vi "BIN_PAQ_UpdateIndexFile.vi"(8 "error in (no error)":errorcluster, 10 "path":path, 11 "TimeRange":T1) -> (0 "error out":errorcluster)   [LabVIEW 2020, in "Sgraph_lib_V1.lvlib" / "DBAL-BIN.lvclass"]
doc: "This method performs a 'read-modify-write' action on the index file that belongs to this table type.\nOnly the line is updated that belongs to the sequence number of this PAQ file.\n\nThe index file enables fast readback for finding the correct file sequence number."
uses:
  DBAL-BIN.lvclass
  controls/DBAL_PAQ_TimeRange.ctl
  DBAL.lvclass
panel:
  out "FileName":string
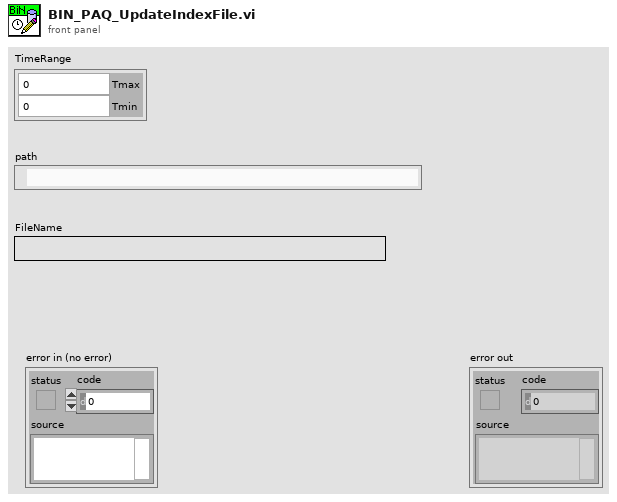
[diagram p1: front panel]
types:
  T1 = typedef "Sgraph_lib_V1.lvlib/DBAL.lvclass/DBAL_PAQ_TimeRange.ctl" = cluster{"Tmax":dbl, "Tmin":dbl}
  T2 = enum16{"open", "replace", "create", "open or create", "replace or create", "replace or create with confirmation"}
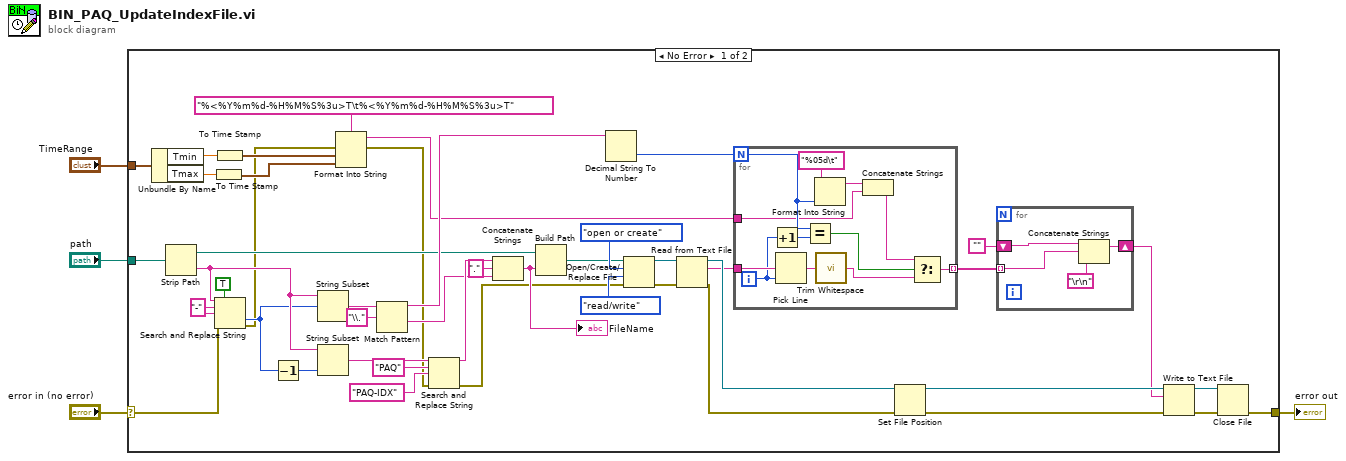
[diagram p0: block diagram]
diagram:
  n1 = case shown="No Error" "error in (no error)" {
    selector: "error in (no error)" -> [w47 w66]
    tunnel: [w19 w66] -> w3
    tunnel: "TimeRange" -> [w15 _]
    tunnel: "path" -> [w49 _]
    frame No Error {
      w48 = "-" ("search string")
      n2 = Unbundle By Name(w15) -> ("Tmin"=w13:dbl, "Tmax"=w14:dbl)
      n3 = Strip Path(path=w49) -> (stripped path=w33:path, name=w45:string)
      n4 = To Time Stamp(1:w14) -> (0:w10:timestamp)
      n5 = To Time Stamp(1:w13) -> (0:w12:timestamp)
      n6 = Search and Replace String(replace all?=TRUE ("replace all? (F)"), input string=w45, search string=w48, replace string=w48, error in=w47) -> (offset past replacement=w44:i32, error out=w9:errorcluster)  [unwired: 3 in, 2 out]
      n7 = Decrement(x=w44) -> (x-1=w41:i32)
      n8 = String Subset(string=w45, offset (0)=w44) -> (substring=w43:string)  [unwired: 1 in]
      n9 = String Subset(string=w45, length (rest)=w41) -> (substring=w39:string)  [unwired: 1 in]
      n10 = Format Into String(format string="%<%Y%m%d-%H%M%S%3u>T\t%<%Y%m%d-%H%M%S%3u>T", error in=w9, w12, w10) -> (resulting string=w5:string, error out=w8:errorcluster)  [unwired: 1 in]
      n11 = Match Pattern(string=w43, regular expression="\\.") -> (before substring=w40:string, after substring=w34:string)  [unwired: 1 in, 2 out]
      n12 = Search and Replace String(input string=w39, search string="PAQ", replace string="PAQ-IDX" ("search string"), error in=w8) -> (result string=w36:string, error out=w25:errorcluster)  [unwired: 4 in, 2 out]
      n13 = Concatenate Strings(w36, "." ("string"), w34) -> (w26:string)
      "FileName" <- w26
      n14 = Build Path(base path=w33, name or relative path=w26) -> (appended path=w30:path)
      n15 = Decimal String To Number(string=w40) -> (number=w27:i32)  [unwired: 2 in, 1 out]
      n16 = Open/Create/Replace File(file path (use dialog)=w30, error in=w25, operation (0:open)=T2."open or create", access (0:read/write)=enum16{"read/write", "read-only", "write-only"}."read/write") -> (refnum out=w28:refnum<file>, error out=w29:errorcluster)  [unwired: 2 in, 1 out]
      n17 = Read from Text File(file (use dialog)=w28, error in=w29) -> (refnum out=w24:refnum<file>, text=w16:string, error out=w7:errorcluster)  [unwired: 2 in, 1 out]
      n18 = for {
        N: w27 -> [w58]
        tunnel: w16 -> [w65]
        tunnel: [w54] -> w6 mode=indexing
        tunnel: w5 -> [w56]
        i -> [w63]
        n19 = Increment(x=w63) -> (x+1=w62:i32)
        n20 = Pick Line(multi-line string=w65, line index=w63) -> (output string=w64:string)  [unwired: 1 in]
        n21 = Equal?(x=w58, y=w62) -> (x = y?=w60:bool)
        n22 = Format Into String(format string="%05d\t", w58) -> (resulting string=w57:string)  [unwired: 2 in, 1 out]
        n23 = call <vilib>:"Trim Whitespace.vi"("string"=w64) -> ("trimmed string"=w61:string)  [unwired: 1 in]
        n24 = Concatenate Strings(w57, w56) -> (w55:string)
        n25 = Select(t=w55, s=w60, f=w61) -> (s? t:f=w54:string)
      }
      n26 = Set File Position(refnum=w24, error in=w7) -> (refnum out=w23:refnum<file>, error out=w22:errorcluster)  [unwired: 2 in]
      n27 = for {
        shift-right: [w50] -> w17
        shift-left: "" -> [w53]
        tunnel: w6 -> [w52] mode=indexing
        n28 = Concatenate Strings(w53, w52, "\r\n") -> (w50:string)
      }
      n29 = Write to Text File(file (use dialog)=w23, text=w17, error in=w22) -> (refnum out=w21:refnum<file>, error out=w20:errorcluster)  [unwired: 1 in, 1 out]
      n30 = Close File(refnum=w21, error in=w20) -> (error out=w19:errorcluster)  [unwired: 1 out]
    }
    frame Error {
    }
  }
  "error out" <- w3
